vi "_measurement_frequencies_from_range_parameters.vi"(0 "Fine range width (Hz)":dbl=40.0, 1 "Fine increment (Hz)":dbl=40.0, 2 "Coarse range width (Hz)":dbl=40.0, 3 "Coarse increment (Hz)":dbl=40.0, 4 "Center frequency (Hz)":dbl=40.0) -> (5 "Measurement frequencies (Hz)":dbl[](array[numeric]), 7 "Fine range start (Hz)":dbl=40.0, 8 "Fine range end (Hz)":dbl=40.0, 9 "Coarse range start (Hz)":dbl=40.0, 10 "Coarse range end (Hz)":dbl=40.0)   [LabVIEW 2020, in "Resonance Curve.lvclass"]
uses:
  Resonance Curve.lvclass
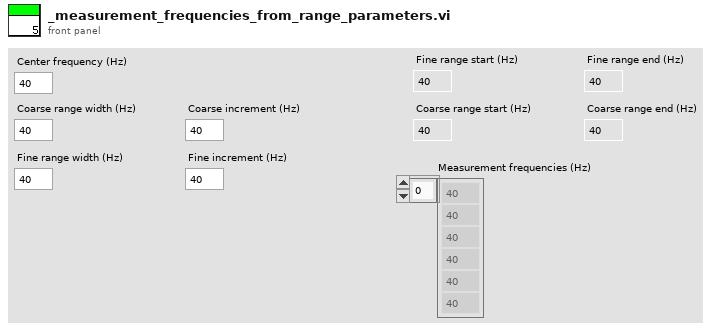
[diagram p1: front panel]
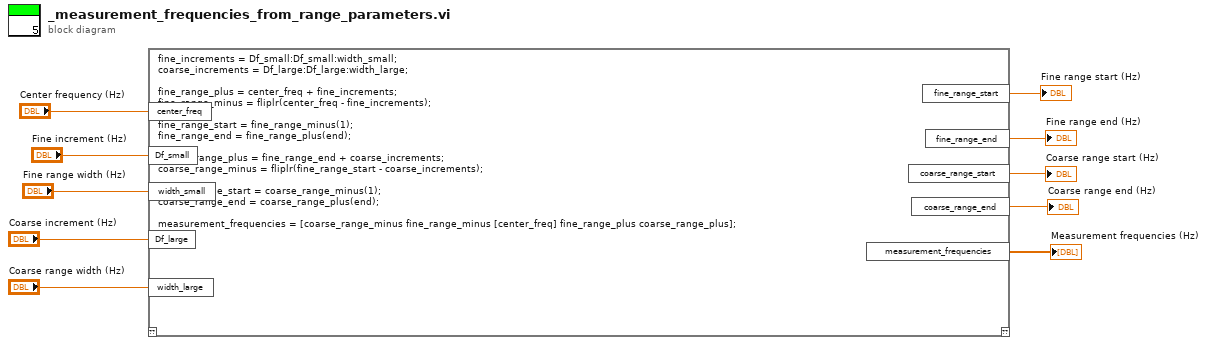
[diagram p0: block diagram]
diagram:
  n1 = script code="fine_increments = Df_small:Df_small:width_small;\ncoarse_increments = Df_large:Df_large:width_large;\n\nfine_range_plus = center_freq + fine_increments;\nfine_range_minus = fliplr(center_freq - fine_increments);\n\nfine_range_start = fine_range_minus(1);\nfine_range_end = fine_range_plus(end);\n\ncoarse_range_plus = fine_range_end + coarse_increments;\ncoarse_range_minus = fliplr(fine_range_start - coarse_increments);\n\ncoarse_range_start = coarse_range_minus(1);\ncoarse_range_end = coarse_range_plus(end);\n\nmeasurement_frequencies = [coarse_range_minus fine_range_minus [center_freq] fine_range_plus coarse_range_plus];"("center_freq"="Center frequency (Hz)", "Df_small"="Fine increment (Hz)", "width_small"="Fine range width (Hz)", "Df_large"="Coarse increment (Hz)", "width_large"="Coarse range width (Hz)") -> ("fine_range_start"=→"Fine range start (Hz)":dbl, "fine_range_end"=→"Fine range end (Hz)":dbl, "coarse_range_start"=→"Coarse range start (Hz)":dbl, "coarse_range_end"=→"Coarse range end (Hz)":dbl, "measurement_frequencies"=→"Measurement frequencies (Hz)":dbl[])  [unwired: 1 in, 1 out]
